vi "Autonomous Independent.vi"() -> ()   [LabVIEW 2016]
doc: "This VI is called when autonomous begins, and will automatically be terminated when autonomous ends. You can carry out timed or sensor driven robot movement independently without needing to return to the caller."
uses:
  <vilib>/Rock Robotics/WPI/Utilities/WPI_GetSetVariantRefNum.vi
  <vilib>/Rock Robotics/Network Tables/NT Write Numeric Array.vi
  <vilib>/Rock Robotics/Network Tables/NT Read String.vi
  <vilib>/Rock Robotics/WPI/RobotDrive/WPI_RobotDriveMecanumDrive_Cartesian.vi
  Encoder Distance.vi
  Cam X.vi
  Cam Y.vi
  Encoder Rate Shooter.vi
panel:
  out "Over Threshold?":bool
  out "High Time (ms)":u32
  out "Over 30 Seconds?":bool
  in  "Shooter Control 2":dbl=0.5
  in  "Shooter Control":dbl=0.5
  out "Current Movement, for debugging":T1 {"Z Joystick Value" scale=-1.0..1.0; "Y Joystick Value" scale=1.0..-1.0; "X Joystick Value" scale=-1.0..1.0}
  in  "Array of robot movements":T2(array[cluster])=[{"X Joystick Value"=-0.010101010101010017, "Y Joystick Value"=0.0, "Z Joystick Value"=0.4574773480918073, "Delay (sec)"=0.0, "Movement Name"=""}, {"X Joystick Value"=0.050505050505050594, "Y Joystick Value"=0.0, "Z Joystick Value"=-0.25616029503917137, "Delay (sec)"=0.0, "Movement Name"=""}] {"Z Joystick Value" scale=-1.0..1.0; "Y Joystick Value" scale=1.0..-1.0; "X Joystick Value" scale=-1.0..1.0}
  # "Be sure to right-click and choose Data Operations>>Make Current Value default if you want to save the array values with the VI"
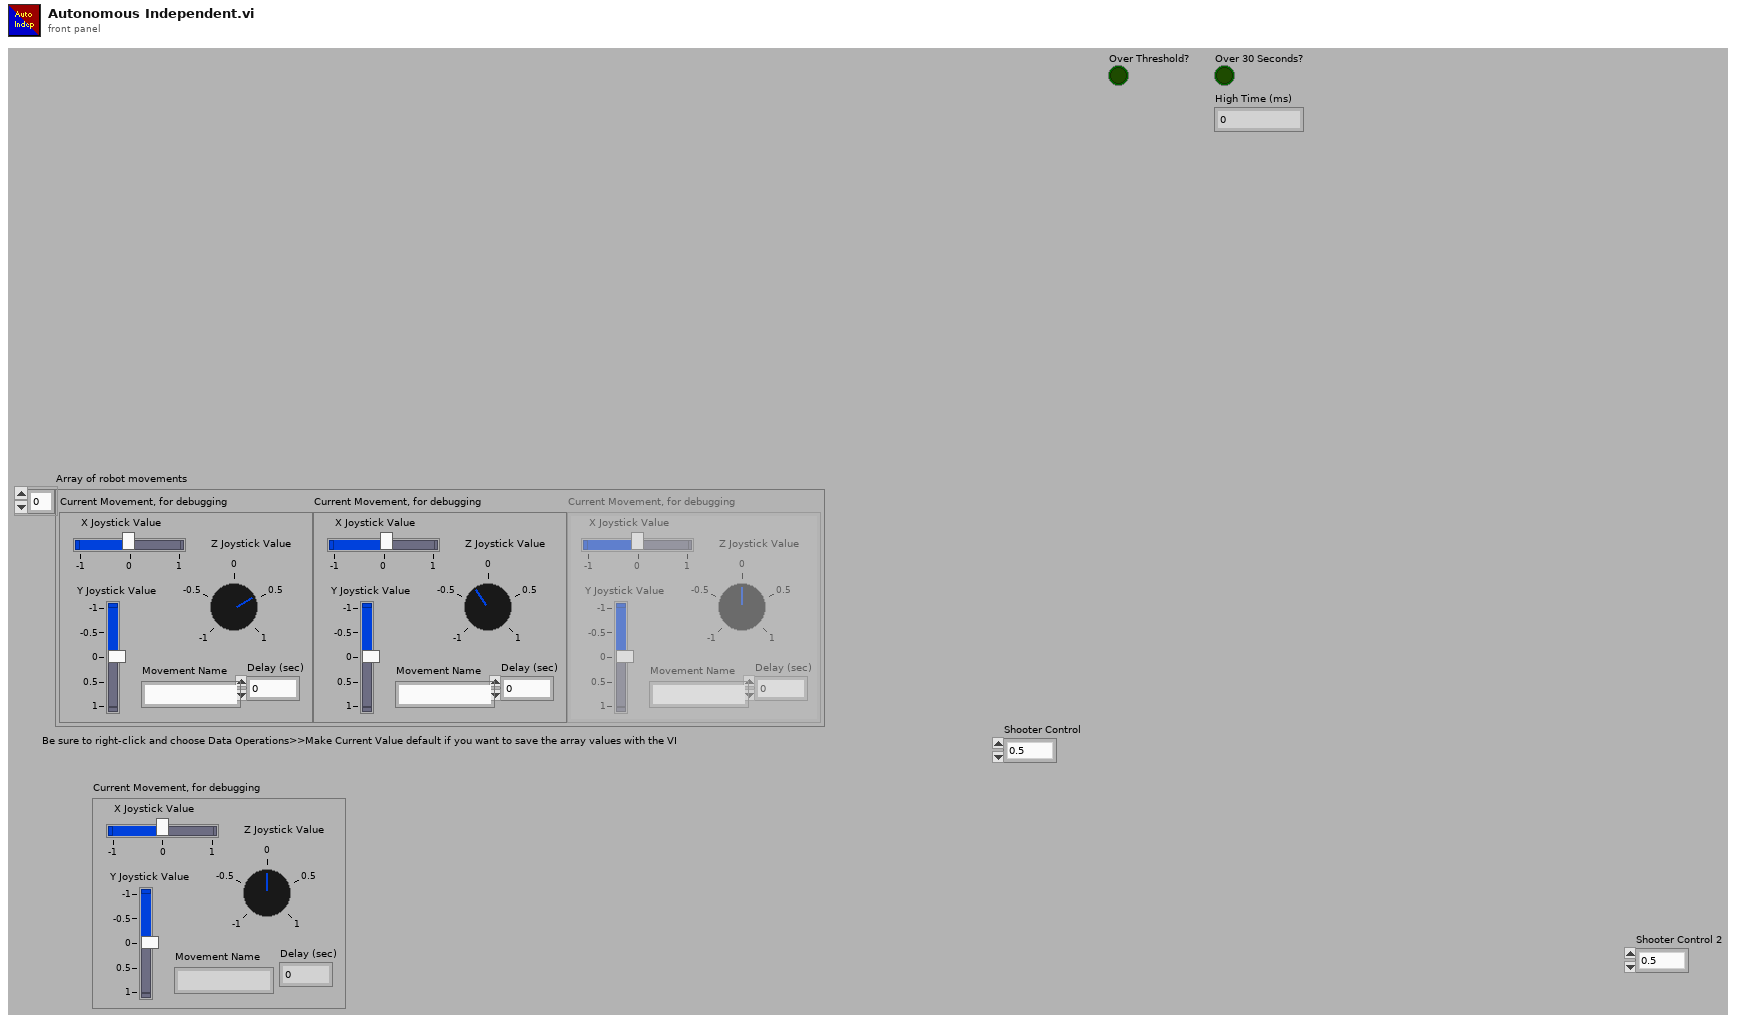
[diagram p1: front panel]
types:
  T1 = cluster{"X Joystick Value":dbl, "Y Joystick Value":dbl, "Z Joystick Value":dbl, "Delay (sec)":dbl, "Movement Name":string}
  T2 = cluster{"X Joystick Value":dbl, "Y Joystick Value":dbl, "Z Joystick Value":dbl, "Delay (sec)":dbl, "Movement Name":string}[]
  T3 = typedef "WPI_JoystickDevRef.ctl" = cluster{"Device":T4}
  T4 = typedef "WPI_JoystickDeviceEnum.ctl" = enum16{"USB 0", "USB 1", "USB 2", "USB 3", "USB 4", "USB 5"}
  T5 = typedef "WPI_RobotDriveDevRef.ctl" = cluster{"DevStatus":errorcluster, "Motors[]":T6[], "Square Inputs":bool, "Max Output":dbl}
  T6 = typedef "WPI_MotorControlDeviceRef.ctl" = cluster{"DeviceStatus":errorcluster, "Type":T7, "PWM":cluster{"PWM Channel":T8, "DeadBand":T9}, "CAN":cluster{"Device Number":u8, "SetOutput VI Ref":variant, "GetOutput VI Ref":variant, "Enable VI Ref":variant, "Disable VI Ref":variant, "Data":variant}, "Invert":bool}
  T7 = typedef "WPI_MotorControlType.ctl" = enum16{"PWM", "CAN"}
  T8 = typedef "FPGA_DIOPWMChannel.ctl" = enum8{"PWM 0", "PWM 1", "PWM 2", "PWM 3", "PWM 4", "PWM 5", "PWM 6", "PWM 7", "PWM 8", "PWM 9", "PWM MXP 0", "PWM MXP 1", "PWM MXP 2", "PWM MXP 3", "PWM MXP 4", "PWM MXP 5", "PWM MXP 6", "PWM MXP 7", "PWM MXP 8", "PWM MXP 9", "Invalid"}
  T9 = typedef "WPI_PWMDeadband.ctl" = cluster{"Name":string, "maxPositivePwm":i32, "minPositivePwm":i32, "centerPwm":i32, "maxNegativePwm":i32, "minNegativePwm":i32, "angularRange":u16}
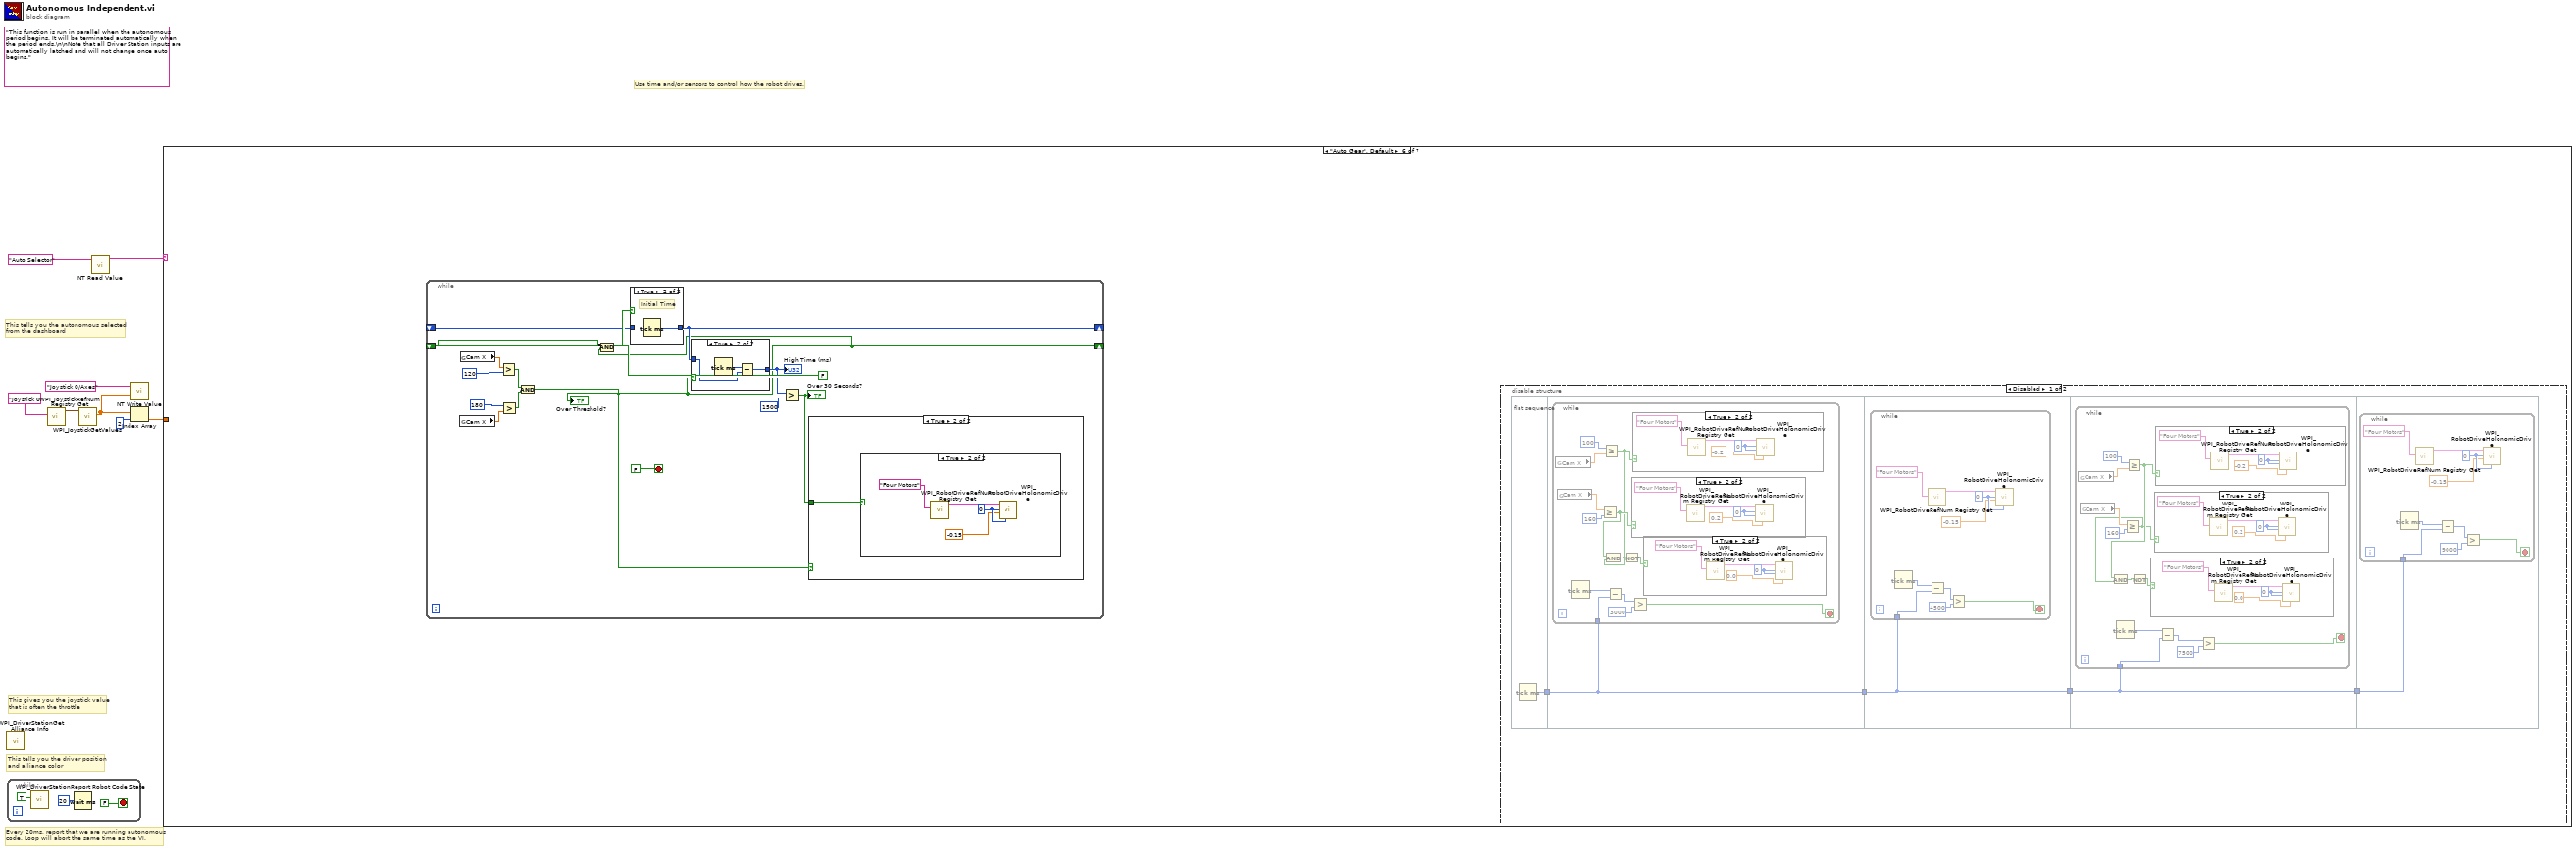
[diagram p0: block diagram]
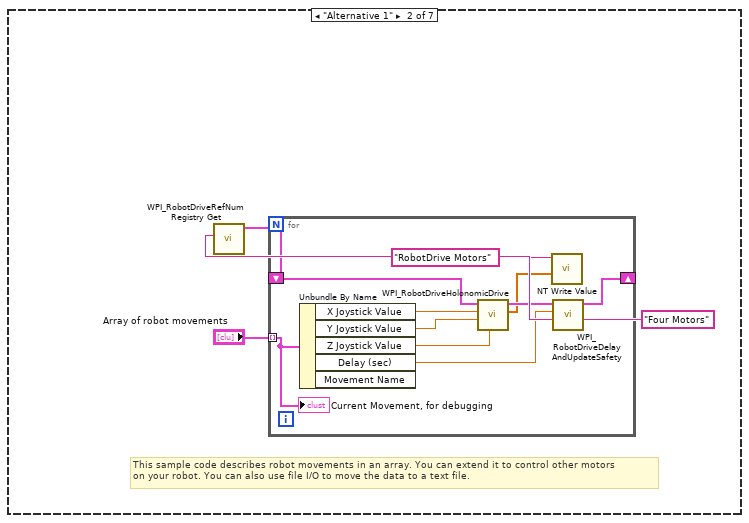
[diagram p3: hidden frame]
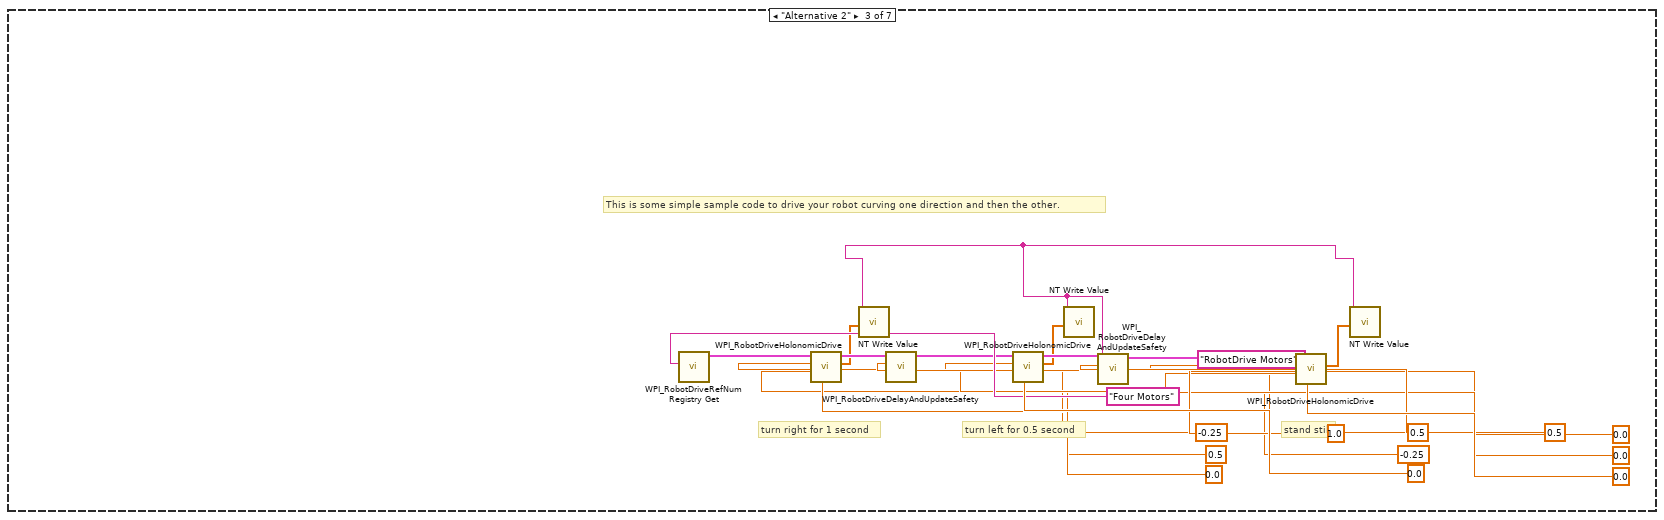
[diagram p4: hidden frame]
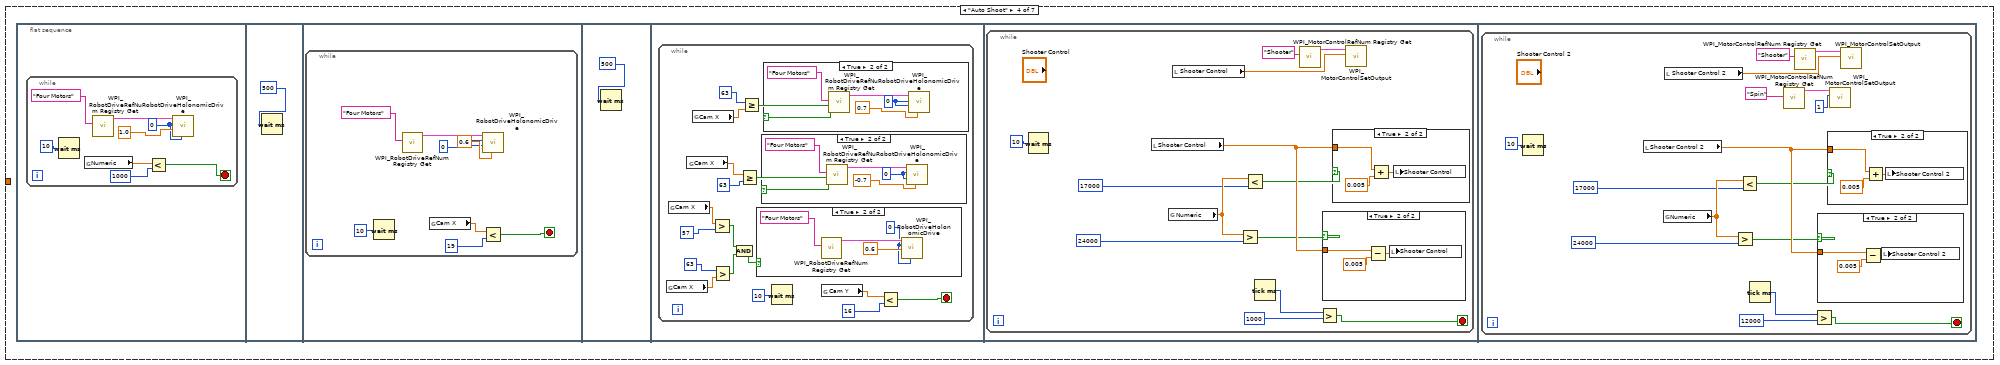
[diagram p5: hidden frame]
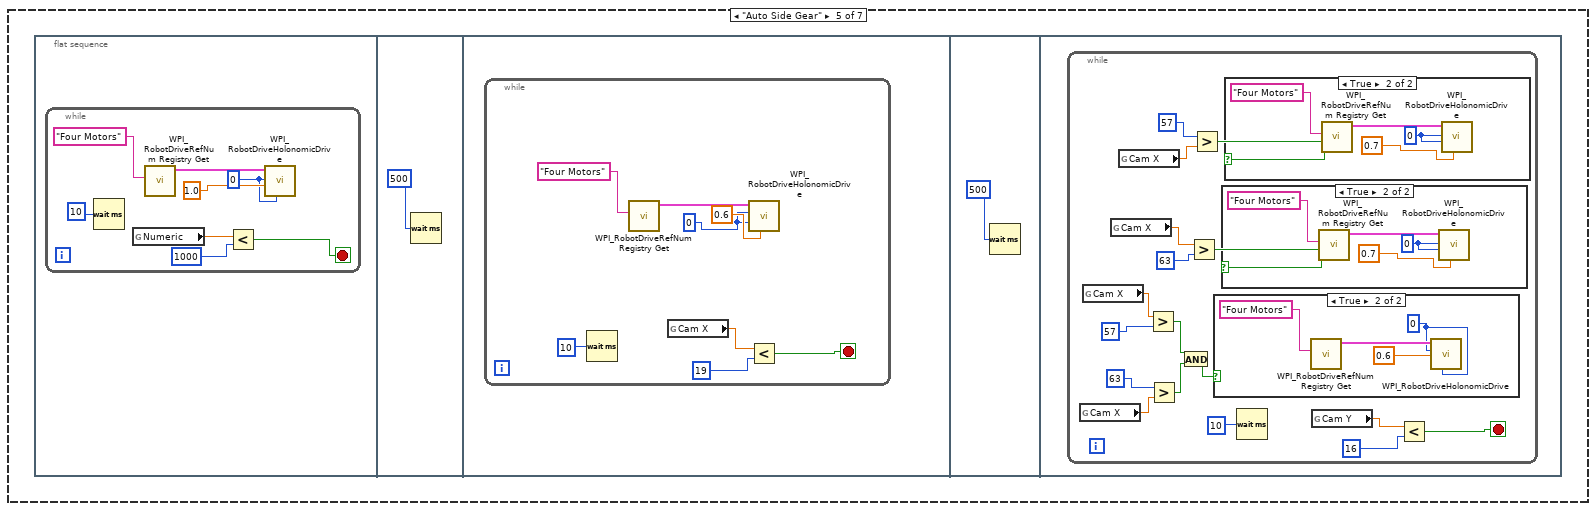
[diagram p13: hidden frame]
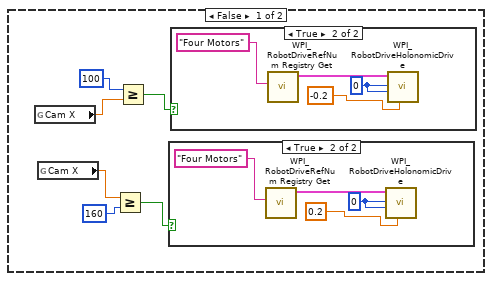
[diagram p17: hidden frame]
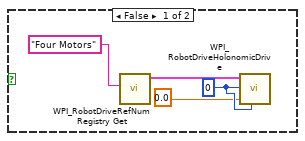
[diagram p20: hidden frame]
diagram:
  (unwired) "This function is run in parallel when the autonomous period begins. It will be terminated automatically when the period ends.\n\nNote that all Driver Station inputs are automatically latched and will not change once auto begins."
  # "This tells you the autonomous selected\nfrom the dashboard"
  # "Every 20ms, report that we are running autonomous\ncode. Loop will abort the same time as the VI."
  # "This gives you the joystick value\nthat is often the throttle"
  # "Use time and/or sensors to control how the robot drives."
  # "This tells you the driver position\nand alliance color"
  n1 = call <vilib>:"WPI_DriverStationGet Alliance Info.vi"() -> ()  [unwired: 12 out]
  n2 = while {
    stop <- FALSE stop-if-true
    n3 = call <vilib>:"WPI_DriverStationReport Robot Code State.vi"("Autonomous"=TRUE) -> ()  [unwired: 10 in, 1 out]
    n4 = Wait (ms)(milliseconds to wait=u32 20) -> ()  [unwired: 1 out]
  }
  n5 = call <vilib>:"WPI_JoystickRefNum Registry Get.vi"("refnum name"="Joystick 0") -> ("JoystickDevRef"=w7:T3)  [unwired: 1 in, 9 out]
  n6 = call <vilib>:"WPI_JoystickGetValues.vi"("JoystickDevRef"=w7) -> ("Axes"=w1:dbl[])  [unwired: 6 in, 4 out]
  n7 = call-poly <vilib>:"NT Read Value.vi"("Name"="Auto Selector") -> ("String"=w4:string)  [unwired: 9 in, 1 out]
  n8 = call-poly <vilib>:"NT Write Value.vi"("Numeric Array"=w1, "Name"="Joystick 0/Axes") -> ()  [unwired: 9 in, 1 out]
  n9 = Index Array(array=w1, index=u32 2 ("milliseconds to wait")) -> (element=w3:dbl)
  n10 = case shown="\"Auto Gear\", Default" w4 {
    tunnel: w3 -> [_ _ _ _ _ _ _]
    frame "hi" {
      # "You can put your main auto here, or you can right-click on the case and make any\nother frame be the default case."
      # "This is the frame that will execute if no selection is made, or if it is not recognized"
    }
    frame "Alternative 1" {
      # "This sample code describes robot movements in an array. You can extend it to control other motors\non your robot. You can also use file I/O to move the data to a text file."
      n11 = call <vilib>:"WPI_RobotDriveRefNum Registry Get.vi"("refnum name"="Four Motors") -> ("RobotDriveDevRef"=w13:T5)  [unwired: 1 in, 9 out]
      n12 = for {
        shift-right: [w22] -> _
        shift-left: w13 -> [w23]
        tunnel: "Array of robot movements" -> [w18] mode=indexing
        n13 = Unbundle By Name(w18) -> ("X Joystick Value"=w21:dbl, "Y Joystick Value"=w20:dbl, "Z Joystick Value"=w17:dbl, "Delay (sec)"=w19:dbl)  [unwired: 1 out]
        n14 = call-poly <vilib>:"WPI_RobotDriveHolonomicDrive.vi"("Rotation"=w17, "Y"=w20, "X"=w21, "RobotDriveDevRef"=w23) -> ("Motor Values"=w15:dbl[], "RobotDriveDevRef"=w24:T5)  [unwired: 5 in, 1 out]
        n15 = call-poly <vilib>:"NT Write Value.vi"("Numeric Array"=w15, "Name"="RobotDrive Motors") -> ()  [unwired: 9 in, 1 out]
        n16 = call <vilib>:"WPI_RobotDriveDelayAndUpdateSafety.vi"("Delay (s)"=w19, "RobotDriveDevRef"=w24) -> ("RobotDriveDevRef 2"=w22:T5)  [unwired: 8 in, 1 out]
        "Current Movement, for debugging" <- w18
      }
    }
    frame "Alternative 2" {
      w25 = "RobotDrive Motors" ("Name")
      # "This is some simple sample code to drive your robot curving one direction and then the other."
      # "stand still"
      # "turn left for 0.5 second"
      # "turn right for 1 second"
      n17 = call <vilib>:"WPI_RobotDriveRefNum Registry Get.vi"("refnum name"="Four Motors") -> ("RobotDriveDevRef"=w42:T5)  [unwired: 1 in, 9 out]
      n18 = call-poly <vilib>:"WPI_RobotDriveHolonomicDrive.vi"("Rotation"=0.0, "Y"=0.5 ("X axis value"), "X"=-0.25 ("X axis value"), "RobotDriveDevRef"=w42) -> ("Motor Values"=w26:dbl[], "RobotDriveDevRef"=w35:T5)  [unwired: 5 in, 1 out]
      n19 = call-poly <vilib>:"NT Write Value.vi"("Numeric Array"=w26, "Name"=w25) -> ()  [unwired: 9 in, 1 out]
      n20 = call <vilib>:"WPI_RobotDriveDelayAndUpdateSafety.vi"("Delay (s)"=1.0, "RobotDriveDevRef"=w35) -> ("RobotDriveDevRef 2"=w36:T5)  [unwired: 8 in, 1 out]
      n21 = call-poly <vilib>:"WPI_RobotDriveHolonomicDrive.vi"("Rotation"=0.0, "Y"=-0.25 ("X axis value"), "X"=0.5 ("X axis value"), "RobotDriveDevRef"=w36) -> ("Motor Values"=w27:dbl[], "RobotDriveDevRef"=w37:T5)  [unwired: 5 in, 1 out]
      n22 = call-poly <vilib>:"NT Write Value.vi"("Numeric Array"=w27, "Name"=w25) -> ()  [unwired: 9 in, 1 out]
      n23 = call <vilib>:"WPI_RobotDriveDelayAndUpdateSafety.vi"("Delay (s)"=0.5, "RobotDriveDevRef"=w37) -> ("RobotDriveDevRef 2"=w38:T5)  [unwired: 8 in, 1 out]
      n24 = call-poly <vilib>:"WPI_RobotDriveHolonomicDrive.vi"("Rotation"=0.0 ("X axis value"), "Y"=0.0 ("X axis value"), "X"=0.0 ("X axis value"), "RobotDriveDevRef"=w38) -> ("Motor Values"=w28:dbl[])  [unwired: 5 in, 2 out]
      n25 = call-poly <vilib>:"NT Write Value.vi"("Numeric Array"=w28, "Name"=w25) -> ()  [unwired: 9 in, 1 out]
    }
    frame "Auto Shoot" {
      n26 = flat-sequence {
        frame #0 {
          n27 = while {
            stop <- w50 stop-if-true
            w46 = 0
            n28 = Wait (ms)(milliseconds to wait=10) -> ()  [unwired: 1 out]
            n29 = global read "Encoder Distance.vi" "Numeric"() -> (w51:dbl)
            n30 = call <vilib>:"WPI_RobotDriveRefNum Registry Get.vi"("refnum name"="Four Motors") -> ("RobotDriveDevRef"=w53:T5)  [unwired: 9 in, 1 out]
            n31 = Less?(x=w51, y=1000) -> (x < y?=w50:bool)
            n32 = call-poly <vilib>:"WPI_RobotDriveHolonomicDrive.vi"("Rotation"=w46, "Y"=1.0, "X"=w46, "RobotDriveDevRef"=w53) -> ()  [unwired: 5 in, 3 out]
          }
        }
        frame #1 {
          n33 = Wait (ms)(milliseconds to wait=500) -> ()  [unwired: 1 out]
        }
        frame #2 {
          n34 = while {
            stop <- w60 stop-if-true
            w55 = 0
            n35 = Wait (ms)(milliseconds to wait=10) -> ()  [unwired: 1 out]
            n36 = call <vilib>:"WPI_RobotDriveRefNum Registry Get.vi"("refnum name"="Four Motors") -> ("RobotDriveDevRef"=w59:T5)  [unwired: 9 in, 1 out]
            n37 = global read "Cam X.vi" "Cam X"() -> (w57:dbl)
            n38 = call-poly <vilib>:"WPI_RobotDriveHolonomicDrive.vi"("Rotation"=0.6, "Y"=w55, "X"=w55, "RobotDriveDevRef"=w59) -> ()  [unwired: 5 in, 3 out]
            n39 = Less?(x=w57, y=19) -> (x < y?=w60:bool)
          }
        }
        frame #3 {
          n40 = Wait (ms)(milliseconds to wait=500) -> ()  [unwired: 1 out]
        }
        frame #4 {
          n41 = while {
            stop <- w76 stop-if-true
            n42 = global read "Cam X.vi" "Cam X"() -> (w65:dbl)
            n43 = global read "Cam X.vi" "Cam X"() -> (w66:dbl)
            n44 = global read "Cam X.vi" "Cam X"() -> (w67:dbl)
            n45 = global read "Cam X.vi" "Cam X"() -> (w68:dbl)
            n46 = Greater?(x=w66, y=57) -> (0:w70:bool)
            n47 = Greater?(x=63, y=w65) -> (0:w69:bool)
            n48 = And(x=w70, y=w69) -> (x .and. y?=w71:bool)
            n49 = Greater Or Equal?(x=w67, y=63) -> (x >= y?=w75:bool)
            n50 = Greater Or Equal?(x=63, y=w68) -> (x >= y?=w79:bool)
            n51 = case shown="True" w71 {
              frame False {
              }
              frame True {
                w81 = 0
                n52 = call <vilib>:"WPI_RobotDriveRefNum Registry Get.vi"("refnum name"="Four Motors") -> ("RobotDriveDevRef"=w84:T5)  [unwired: 9 in, 1 out]
                n53 = call-poly <vilib>:"WPI_RobotDriveHolonomicDrive.vi"("Rotation"=w81, "Y"=0.6, "X"=w81, "RobotDriveDevRef"=w84) -> ()  [unwired: 5 in, 3 out]
              }
            }
            n54 = case shown="True" w75 {
              frame False {
              }
              frame True {
                w85 = 0
                n55 = call <vilib>:"WPI_RobotDriveRefNum Registry Get.vi"("refnum name"="Four Motors") -> ("RobotDriveDevRef"=w88:T5)  [unwired: 9 in, 1 out]
                n56 = call-poly <vilib>:"WPI_RobotDriveHolonomicDrive.vi"("Rotation"=-0.7, "Y"=w85, "X"=w85, "RobotDriveDevRef"=w88) -> ()  [unwired: 5 in, 3 out]
              }
            }
            n57 = case shown="True" w79 {
              frame False {
              }
              frame True {
                w89 = 0
                n58 = call <vilib>:"WPI_RobotDriveRefNum Registry Get.vi"("refnum name"="Four Motors") -> ("RobotDriveDevRef"=w92:T5)  [unwired: 9 in, 1 out]
                n59 = call-poly <vilib>:"WPI_RobotDriveHolonomicDrive.vi"("Rotation"=0.7, "Y"=w89, "X"=w89, "RobotDriveDevRef"=w92) -> ()  [unwired: 5 in, 3 out]
              }
            }
            n60 = Wait (ms)(milliseconds to wait=10) -> ()  [unwired: 1 out]
            n61 = global read "Cam Y.vi" "Cam Y"() -> (w64:dbl)
            n62 = Less?(x=w64, y=16) -> (x < y?=w76:bool)
          }
        }
        frame #5 {
          n63 = while {
            stop <- w94 stop-if-true
            n64 = Wait (ms)(milliseconds to wait=10) -> ()  [unwired: 1 out]
            n65 = local read "Shooter Control"() -> (w105:dbl)
            n66 = global read "Encoder Rate Shooter.vi" "Numeric"() -> (w102:dbl)
            n67 = local read "Shooter Control"() -> (w97:dbl)
            n68 = Greater?(x=w102, y=24000) -> (0:w104:bool)
            n69 = Less?(x=w102, y=17000) -> (x < y?=w103:bool)
            n70 = Tick Count (ms)() -> (millisecond timer value=w96:u32)
            n71 = call <vilib>:"WPI_MotorControlRefNum Registry Get.vi"("refnum name"="Shooter") -> ("MotorControlDevRef"=w99:T6)  [unwired: 9 in, 1 out]
            n72 = Greater?(x=w96, y=1000) -> (0:w94:bool)
            n73 = case shown="True" w104 {
              tunnel: w105 -> [_ w106]
              frame False {
              }
              frame True {
                n74 = Subtract(x=w106, y=0.005) -> (x-y=w107:dbl)
                n75 = local write "Shooter Control"(w107) -> ()
              }
            }
            n76 = case shown="True" w103 {
              tunnel: w105 -> [_ w109]
              frame False {
              }
              frame True {
                n77 = Add(x=w109, y=0.005) -> (x+y=w110:dbl)
                n78 = local write "Shooter Control"(w110) -> ()
              }
            }
            n79 = call <vilib>:"WPI_MotorControlSetOutput.vi"("Output"=w97, "MotorControlDevRef"=w99) -> ()  [unwired: 7 in, 3 out]
          }
        }
        frame #6 {
          n80 = while {
            stop <- w113 stop-if-true
            n81 = Wait (ms)(milliseconds to wait=10) -> ()  [unwired: 1 out]
            n82 = local read "Shooter Control 2"() -> (w127:dbl)
            n83 = global read "Encoder Rate Shooter.vi" "Numeric"() -> (w124:dbl)
            n84 = local read "Shooter Control 2"() -> (w119:dbl)
            n85 = Greater?(x=w124, y=24000) -> (0:w126:bool)
            n86 = Less?(x=w124, y=17000) -> (x < y?=w125:bool)
            n87 = Tick Count (ms)() -> (millisecond timer value=w115:u32)
            n88 = call <vilib>:"WPI_MotorControlRefNum Registry Get.vi"("refnum name"="Spin") -> ("MotorControlDevRef"=w117:T6)  [unwired: 9 in, 1 out]
            n89 = call <vilib>:"WPI_MotorControlRefNum Registry Get.vi"("refnum name"="Shooter") -> ("MotorControlDevRef"=w121:T6)  [unwired: 9 in, 1 out]
            n90 = Greater?(x=w115, y=12000) -> (0:w113:bool)
            n91 = case shown="True" w126 {
              tunnel: w127 -> [_ w128]
              frame False {
              }
              frame True {
                n92 = Subtract(x=w128, y=0.005) -> (x-y=w129:dbl)
                n93 = local write "Shooter Control 2"(w129) -> ()
              }
            }
            n94 = case shown="True" w125 {
              tunnel: w127 -> [_ w131]
              frame False {
              }
              frame True {
                n95 = Add(x=w131, y=0.005) -> (x+y=w132:dbl)
                n96 = local write "Shooter Control 2"(w132) -> ()
              }
            }
            n97 = call <vilib>:"WPI_MotorControlSetOutput.vi"("Output"=1, "MotorControlDevRef"=w117) -> ()  [unwired: 7 in, 3 out]
            n98 = call <vilib>:"WPI_MotorControlSetOutput.vi"("Output"=w119, "MotorControlDevRef"=w121) -> ()  [unwired: 7 in, 3 out]
          }
        }
      }
    }
    frame "Auto Side Gear" {
      n99 = flat-sequence {
        frame #0 {
          n100 = while {
            stop <- w137 stop-if-true
            w135 = 0
            n101 = Wait (ms)(milliseconds to wait=10) -> ()  [unwired: 1 out]
            n102 = global read "Encoder Distance.vi" "Numeric"() -> (w138:dbl)
            n103 = call <vilib>:"WPI_RobotDriveRefNum Registry Get.vi"("refnum name"="Four Motors") -> ("RobotDriveDevRef"=w141:T5)  [unwired: 9 in, 1 out]
            n104 = Less?(x=w138, y=1000) -> (x < y?=w137:bool)
            n105 = call-poly <vilib>:"WPI_RobotDriveHolonomicDrive.vi"("Rotation"=w135, "Y"=1.0, "X"=w135, "RobotDriveDevRef"=w141) -> ()  [unwired: 5 in, 3 out]
          }
        }
        frame #1 {
          n106 = Wait (ms)(milliseconds to wait=500) -> ()  [unwired: 1 out]
        }
        frame #2 {
          n107 = while {
            stop <- w148 stop-if-true
            w143 = 0
            n108 = Wait (ms)(milliseconds to wait=10) -> ()  [unwired: 1 out]
            n109 = call <vilib>:"WPI_RobotDriveRefNum Registry Get.vi"("refnum name"="Four Motors") -> ("RobotDriveDevRef"=w147:T5)  [unwired: 9 in, 1 out]
            n110 = global read "Cam X.vi" "Cam X"() -> (w145:dbl)
            n111 = call-poly <vilib>:"WPI_RobotDriveHolonomicDrive.vi"("Rotation"=0.6, "Y"=w143, "X"=w143, "RobotDriveDevRef"=w147) -> ()  [unwired: 5 in, 3 out]
            n112 = Less?(x=w145, y=19) -> (x < y?=w148:bool)
          }
        }
        frame #3 {
          n113 = Wait (ms)(milliseconds to wait=500) -> ()  [unwired: 1 out]
        }
        frame #4 {
          n114 = while {
            stop <- w164 stop-if-true
            n115 = global read "Cam X.vi" "Cam X"() -> (w153:dbl)
            n116 = global read "Cam X.vi" "Cam X"() -> (w154:dbl)
            n117 = global read "Cam X.vi" "Cam X"() -> (w155:dbl)
            n118 = global read "Cam X.vi" "Cam X"() -> (w156:dbl)
            n119 = Greater?(x=w154, y=57) -> (0:w158:bool)
            n120 = Greater?(x=63, y=w153) -> (0:w157:bool)
            n121 = And(x=w158, y=w157) -> (x .and. y?=w159:bool)
            n122 = Greater?(x=w155, y=63) -> (0:w163:bool)
            n123 = Greater?(x=57, y=w156) -> (0:w167:bool)
            n124 = case shown="True" w159 {
              frame False {
              }
              frame True {
                w169 = 0
                n125 = call <vilib>:"WPI_RobotDriveRefNum Registry Get.vi"("refnum name"="Four Motors") -> ("RobotDriveDevRef"=w172:T5)  [unwired: 9 in, 1 out]
                n126 = call-poly <vilib>:"WPI_RobotDriveHolonomicDrive.vi"("Rotation"=w169, "Y"=0.6, "X"=w169, "RobotDriveDevRef"=w172) -> ()  [unwired: 5 in, 3 out]
              }
            }
            n127 = case shown="True" w163 {
              frame False {
              }
              frame True {
                w173 = 0
                n128 = call <vilib>:"WPI_RobotDriveRefNum Registry Get.vi"("refnum name"="Four Motors") -> ("RobotDriveDevRef"=w176:T5)  [unwired: 9 in, 1 out]
                n129 = call-poly <vilib>:"WPI_RobotDriveHolonomicDrive.vi"("Rotation"=0.7, "Y"=w173, "X"=w173, "RobotDriveDevRef"=w176) -> ()  [unwired: 5 in, 3 out]
              }
            }
            n130 = case shown="True" w167 {
              frame False {
              }
              frame True {
                w177 = 0
                n131 = call <vilib>:"WPI_RobotDriveRefNum Registry Get.vi"("refnum name"="Four Motors") -> ("RobotDriveDevRef"=w180:T5)  [unwired: 9 in, 1 out]
                n132 = call-poly <vilib>:"WPI_RobotDriveHolonomicDrive.vi"("Rotation"=0.7, "Y"=w177, "X"=w177, "RobotDriveDevRef"=w180) -> ()  [unwired: 5 in, 3 out]
              }
            }
            n133 = Wait (ms)(milliseconds to wait=10) -> ()  [unwired: 1 out]
            n134 = global read "Cam Y.vi" "Cam Y"() -> (w152:dbl)
            n135 = Less?(x=w152, y=16) -> (x < y?=w164:bool)
          }
        }
      }
    }
    frame "Auto Gear", Default {
      n136 = while {
        shift-right: [w194] -> _
        shift-left: _ -> [w195]
        shift-right: [w182] -> _
        shift-left: FALSE -> [w191]
        stop <- FALSE stop-if-true
        n137 = global read "Cam X.vi" "Cam X"() -> (w189:dbl)
        n138 = global read "Cam X.vi" "Cam X"() -> (w190:dbl)
        n139 = Greater?(x=w190, y=120) -> (0:w187:bool)
        n140 = Greater?(x=180, y=w189) -> (0:w188:bool)
        n141 = And(x=w187, y=w188) -> (x .and. y?=w182:bool)
        "Over Threshold?" <- w182
        n142 = Compound Arithmetic op=AND(invert w191, w182) -> (w196:bool)
        n143 = case shown="True" w196 {
          tunnel: [w224 w225] -> w194
          tunnel: w195 -> [w224 _]
          frame False {
          }
          frame True {
            # "Initial Time"
            n144 = Tick Count (ms)() -> (millisecond timer value=w225:u32)
          }
        }
        n145 = case shown="True" w182 {
          tunnel: w194 -> [_ w222]
          tunnel: [u32 0 w221] -> w193
          frame False {
          }
          frame True {
            n146 = Tick Count (ms)() -> (millisecond timer value=w223:u32)
            n147 = Subtract(x=w223, y=w222) -> (x-y=w221:u32)
          }
        }
        "High Time (ms)" <- w193
        n148 = Greater?(x=w193, y=u32 1500) -> (0:w183:bool)
        "Over 30 Seconds?" <- w183
        n149 = case shown="True" w182 {
          tunnel: w183 -> [_ w211]
          frame False {
            n150 = global read "Cam X.vi" "Cam X"() -> (w200:dbl)
            n151 = global read "Cam X.vi" "Cam X"() -> (w199:dbl)
            n152 = Greater Or Equal?(x=w199, y=160) -> (x >= y?=w198:bool)
            n153 = Greater Or Equal?(x=100, y=w200) -> (x >= y?=w197:bool)
            n154 = case shown="True" w198 {
              frame False {
              }
              frame True {
                w203 = 0
                n155 = call <vilib>:"WPI_RobotDriveRefNum Registry Get.vi"("refnum name"="Four Motors") -> ("RobotDriveDevRef"=w206:T5)  [unwired: 9 in, 1 out]
                n156 = call-poly <vilib>:"WPI_RobotDriveHolonomicDrive.vi"("Rotation"=0.2, "Y"=w203, "X"=w203, "RobotDriveDevRef"=w206) -> ()  [unwired: 5 in, 3 out]
              }
            }
            n157 = case shown="True" w197 {
              frame False {
              }
              frame True {
                w207 = 0
                n158 = call <vilib>:"WPI_RobotDriveRefNum Registry Get.vi"("refnum name"="Four Motors") -> ("RobotDriveDevRef"=w210:T5)  [unwired: 9 in, 1 out]
                n159 = call-poly <vilib>:"WPI_RobotDriveHolonomicDrive.vi"("Rotation"=-0.2, "Y"=w207, "X"=w207, "RobotDriveDevRef"=w210) -> ()  [unwired: 5 in, 3 out]
              }
            }
          }
          frame True {
            n160 = case shown="True" w211 {
              frame False {
                w213 = 0
                n161 = call <vilib>:"WPI_RobotDriveRefNum Registry Get.vi"("refnum name"="Four Motors") -> ("RobotDriveDevRef"=w215:T5)  [unwired: 9 in, 1 out]
                n162 = call-poly <vilib>:"WPI_RobotDriveHolonomicDrive.vi"("Rotation"=w213, "Y"=0.0, "X"=w213, "RobotDriveDevRef"=w215) -> ()  [unwired: 5 in, 3 out]
              }
              frame True {
                w217 = 0
                n163 = call <vilib>:"WPI_RobotDriveRefNum Registry Get.vi"("refnum name"="Four Motors") -> ("RobotDriveDevRef"=w219:T5)  [unwired: 9 in, 1 out]
                n164 = call-poly <vilib>:"WPI_RobotDriveHolonomicDrive.vi"("Rotation"=w217, "Y"=-0.15, "X"=w217, "RobotDriveDevRef"=w219) -> ()  [unwired: 5 in, 3 out]
              }
            }
          }
        }
      }
      n165 = disable-structure shown="Disabled" {
        frame Disabled {
          n166 = flat-sequence {
            tunnel: [w230] -> w229
            tunnel: w229 -> [w231]
            tunnel: [w231] -> w228
            tunnel: w228 -> [w257]
            tunnel: [w257] -> w227
            tunnel: w227 -> [w267]
            tunnel: [w267] -> w226
            tunnel: w226 -> [w293]
            frame #0 {
              n167 = Tick Count (ms)() -> (millisecond timer value=w230:u32)
            }
            frame #1 {
              n168 = while {
                tunnel: w231 -> [w232]
                stop <- w238 stop-if-true
                n169 = global read "Cam X.vi" "Cam X"() -> (w242:dbl)
                n170 = global read "Cam X.vi" "Cam X"() -> (w241:dbl)
                n171 = Tick Count (ms)() -> (millisecond timer value=w233:u32)
                n172 = Greater Or Equal?(x=w241, y=160) -> (x >= y?=w237:bool)
                n173 = Greater Or Equal?(x=100, y=w242) -> (x >= y?=w236:bool)
                n174 = And(x=w237, y=w236) -> (x .and. y?=w234:bool)
                n175 = Subtract(x=w233, y=w232) -> (x-y=w240:u32)
                n176 = Not(x=w234) -> (.not. x?=w235:bool)
                n177 = case shown="True" w237 {
                  frame False {
                  }
                  frame True {
                    w249 = 0
                    n178 = call <vilib>:"WPI_RobotDriveRefNum Registry Get.vi"("refnum name"="Four Motors") -> ("RobotDriveDevRef"=w252:T5)  [unwired: 9 in, 1 out]
                    n179 = call-poly <vilib>:"WPI_RobotDriveHolonomicDrive.vi"("Rotation"=0.2, "Y"=w249, "X"=w249, "RobotDriveDevRef"=w252) -> ()  [unwired: 5 in, 3 out]
                  }
                }
                n180 = Greater?(x=w240, y=3000) -> (0:w238:bool)
                n181 = case shown="True" w236 {
                  frame False {
                  }
                  frame True {
                    w253 = 0
                    n182 = call <vilib>:"WPI_RobotDriveRefNum Registry Get.vi"("refnum name"="Four Motors") -> ("RobotDriveDevRef"=w256:T5)  [unwired: 9 in, 1 out]
                    n183 = call-poly <vilib>:"WPI_RobotDriveHolonomicDrive.vi"("Rotation"=-0.2, "Y"=w253, "X"=w253, "RobotDriveDevRef"=w256) -> ()  [unwired: 5 in, 3 out]
                  }
                }
                n184 = case shown="True" w235 {
                  frame False {
                  }
                  frame True {
                    w245 = 0
                    n185 = call <vilib>:"WPI_RobotDriveRefNum Registry Get.vi"("refnum name"="Four Motors") -> ("RobotDriveDevRef"=w248:T5)  [unwired: 9 in, 1 out]
                    n186 = call-poly <vilib>:"WPI_RobotDriveHolonomicDrive.vi"("Rotation"=0.0, "Y"=w245, "X"=w245, "RobotDriveDevRef"=w248) -> ()  [unwired: 5 in, 3 out]
                  }
                }
              }
            }
            frame #2 {
              n187 = while {
                tunnel: w257 -> [w258]
                stop <- w260 stop-if-true
                w264 = 0
                n188 = Tick Count (ms)() -> (millisecond timer value=w259:u32)
                n189 = call <vilib>:"WPI_RobotDriveRefNum Registry Get.vi"("refnum name"="Four Motors") -> ("RobotDriveDevRef"=w266:T5)  [unwired: 9 in, 1 out]
                n190 = Subtract(x=w259, y=w258) -> (x-y=w261:u32)
                n191 = Greater?(x=w261, y=4500) -> (0:w260:bool)
                n192 = call-poly <vilib>:"WPI_RobotDriveHolonomicDrive.vi"("Rotation"=w264, "Y"=-0.15, "X"=w264, "RobotDriveDevRef"=w266) -> ()  [unwired: 5 in, 3 out]
              }
            }
            frame #3 {
              n193 = while {
                tunnel: w267 -> [w268]
                stop <- w274 stop-if-true
                n194 = global read "Cam X.vi" "Cam X"() -> (w278:dbl)
                n195 = global read "Cam X.vi" "Cam X"() -> (w277:dbl)
                n196 = Tick Count (ms)() -> (millisecond timer value=w269:u32)
                n197 = Greater Or Equal?(x=w277, y=160) -> (x >= y?=w270:bool)
                n198 = Greater Or Equal?(x=100, y=w278) -> (x >= y?=w271:bool)
                n199 = And(x=w271, y=w270) -> (x .and. y?=w272:bool)
                n200 = Not(x=w272) -> (.not. x?=w273:bool)
                n201 = case shown="True" w273 {
                  frame False {
                  }
                  frame True {
                    w281 = 0
                    n202 = call <vilib>:"WPI_RobotDriveRefNum Registry Get.vi"("refnum name"="Four Motors") -> ("RobotDriveDevRef"=w284:T5)  [unwired: 9 in, 1 out]
                    n203 = call-poly <vilib>:"WPI_RobotDriveHolonomicDrive.vi"("Rotation"=0.0, "Y"=w281, "X"=w281, "RobotDriveDevRef"=w284) -> ()  [unwired: 5 in, 3 out]
                  }
                }
                n204 = case shown="True" w270 {
                  frame False {
                  }
                  frame True {
                    w285 = 0
                    n205 = call <vilib>:"WPI_RobotDriveRefNum Registry Get.vi"("refnum name"="Four Motors") -> ("RobotDriveDevRef"=w288:T5)  [unwired: 9 in, 1 out]
                    n206 = call-poly <vilib>:"WPI_RobotDriveHolonomicDrive.vi"("Rotation"=0.2, "Y"=w285, "X"=w285, "RobotDriveDevRef"=w288) -> ()  [unwired: 5 in, 3 out]
                  }
                }
                n207 = case shown="True" w271 {
                  frame False {
                  }
                  frame True {
                    w289 = 0
                    n208 = call <vilib>:"WPI_RobotDriveRefNum Registry Get.vi"("refnum name"="Four Motors") -> ("RobotDriveDevRef"=w292:T5)  [unwired: 9 in, 1 out]
                    n209 = call-poly <vilib>:"WPI_RobotDriveHolonomicDrive.vi"("Rotation"=-0.2, "Y"=w289, "X"=w289, "RobotDriveDevRef"=w292) -> ()  [unwired: 5 in, 3 out]
                  }
                }
                n210 = Subtract(x=w269, y=w268) -> (x-y=w276:u32)
                n211 = Greater?(x=w276, y=7500) -> (0:w274:bool)
              }
            }
            frame #4 {
              n212 = while {
                tunnel: w293 -> [w294]
                stop <- w296 stop-if-true
                w300 = 0
                n213 = Tick Count (ms)() -> (millisecond timer value=w295:u32)
                n214 = call <vilib>:"WPI_RobotDriveRefNum Registry Get.vi"("refnum name"="Four Motors") -> ("RobotDriveDevRef"=w302:T5)  [unwired: 9 in, 1 out]
                n215 = Subtract(x=w295, y=w294) -> (x-y=w297:u32)
                n216 = Greater?(x=w297, y=9000) -> (0:w296:bool)
                n217 = call-poly <vilib>:"WPI_RobotDriveHolonomicDrive.vi"("Rotation"=w300, "Y"=-0.15, "X"=w300, "RobotDriveDevRef"=w302) -> ()  [unwired: 5 in, 3 out]
              }
            }
          }
        }
        frame Enabled {
        }
      }
    }
    frame "Follow target" {
      n218 = while {
        stop <- FALSE stop-if-true
        n219 = global read "Cam X.vi" "Cam X"() -> (w307:dbl)
        n220 = global read "Cam X.vi" "Cam X"() -> (w308:dbl)
        n221 = global read "Cam X.vi" "Cam X"() -> (w309:dbl)
        n222 = global read "Cam X.vi" "Cam X"() -> (w310:dbl)
        n223 = Greater?(x=w308, y=245) -> (0:w312:bool)
        n224 = Greater?(x=265, y=w307) -> (0:w311:bool)
        n225 = And(x=w312, y=w311) -> (x .and. y?=w303:bool)
        n226 = Greater Or Equal?(x=w309, y=265) -> (x >= y?=w304:bool)
        n227 = Greater Or Equal?(x=245, y=w310) -> (x >= y?=w305:bool)
        n228 = Wait (ms)(milliseconds to wait=10) -> ()  [unwired: 1 out]
        n229 = case shown="True" w304 {
          frame False {
          }
          frame True {
            w322 = 0
            n230 = call <vilib>:"WPI_RobotDriveRefNum Registry Get.vi"("refnum name"="Four Motors") -> ("RobotDriveDevRef"=w325:T5)  [unwired: 9 in, 1 out]
            n231 = call-poly <vilib>:"WPI_RobotDriveHolonomicDrive.vi"("Rotation"=-0.7, "Y"=w322, "X"=w322, "RobotDriveDevRef"=w325) -> ()  [unwired: 5 in, 3 out]
          }
        }
        n232 = case shown="True" w305 {
          frame False {
          }
          frame True {
            w326 = 0
            n233 = call <vilib>:"WPI_RobotDriveRefNum Registry Get.vi"("refnum name"="Four Motors") -> ("RobotDriveDevRef"=w329:T5)  [unwired: 9 in, 1 out]
            n234 = call-poly <vilib>:"WPI_RobotDriveHolonomicDrive.vi"("Rotation"=0.7, "Y"=w326, "X"=w326, "RobotDriveDevRef"=w329) -> ()  [unwired: 5 in, 3 out]
          }
        }
        n235 = case shown="True" w303 {
          frame False {
          }
          frame True {
            w318 = 0
            n236 = call <vilib>:"WPI_RobotDriveRefNum Registry Get.vi"("refnum name"="Four Motors") -> ("RobotDriveDevRef"=w321:T5)  [unwired: 9 in, 1 out]
            n237 = call-poly <vilib>:"WPI_RobotDriveHolonomicDrive.vi"("Rotation"=w318, "Y"=0.6, "X"=w318, "RobotDriveDevRef"=w321) -> ()  [unwired: 5 in, 3 out]
          }
        }
      }
    }
  }
